vi "Reset Modules.vi"(8 "error in (no error)":errorcluster, 10 "Modules to Reset (All F:None)":bool[](array[boolean])=[FALSE, FALSE, FALSE, FALSE], 11 "VISA Resource Name":refnum<visa-resource-name>) -> (0 "error out":errorcluster, 3 "VISA Resource Name Out":refnum<visa-resource-name>)   [LabVIEW 2016, in "Agilent 34970.lvlib"]
doc: "This VI allows you to reset one or more modules to their power-on states."
uses:
  Agilent 34970.lvlib
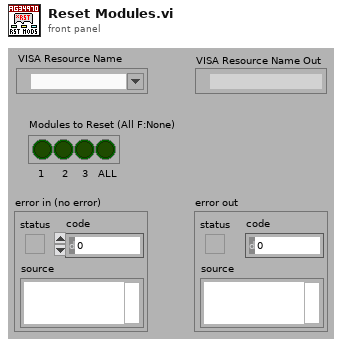
[diagram p1: front panel]
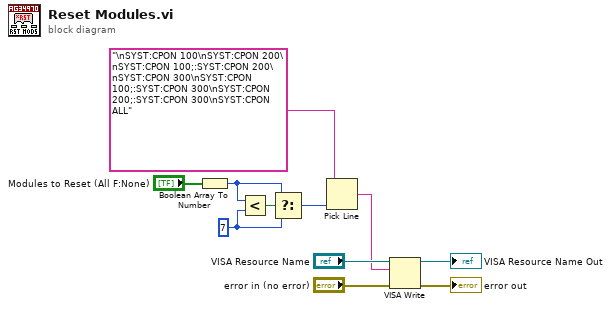
[diagram p0: block diagram]
diagram:
  w9 = u32 7 ("y")
  n1 = Boolean Array To Number(Boolean array="Modules to Reset (All F:None)") -> (number=w10:u32)
  n2 = Less?(x=w10, y=w9) -> (x < y?=w11:bool)
  n3 = Select(t=w10, s=w11, f=w9) -> (s? t:f=w8:u32)
  n4 = Pick Line(multi-line string="\nSYST:CPON 100\nSYST:CPON 200\nSYST:CPON 100;:SYST:CPON 200\nSYST:CPON 300\nSYST:CPON 100;:SYST:CPON 300\nSYST:CPON 200;:SYST:CPON 300\nSYST:CPON ALL" ("string (\"\")"), line index=w8) -> (output string=w2:string)  [unwired: 1 in]
  n5 = VISA Write(VISA resource name="VISA Resource Name", write buffer=w2, error in (no error)="error in (no error)") -> (VISA resource name out=→"VISA Resource Name Out":refnum<visa-resource-name>, error out=→"error out":errorcluster)  [unwired: 1 out]
